vi "SaveTCInfo.vi"(8 "error in (no error)":errorcluster, 10 "Save":bool=TRUE, 11 "TestSeqClass.lvclass":refnum<class "TestSeqClass.lvclass">) -> (0 "error out":errorcluster, 3 "TestSeqClass out":refnum<class "TestSeqClass.lvclass">)   [LabVIEW 2017, in "TestSeqClass.lvclass"]
uses:
  TestSeqClass.lvclass
  Typedef/TestTypeSelect.ctl
  TestMeasureStep/TypeDef/TesstepType.ctl
  Typedef/TestStatus.ctl
  TestMeasureStep/TestMeasureStep.lvclass
  TestMeasureStep/TestMeasureStep.lvclass/TestMeasureStep.ctl
  GUIHandler_Main/GUI_Handler_Main.lvclass
  GUIHandler/GUI_Handler_Seq.lvclass
panel:
  in  "TestType":T1
  in  "ResultListBox":i32(listbox)=-1
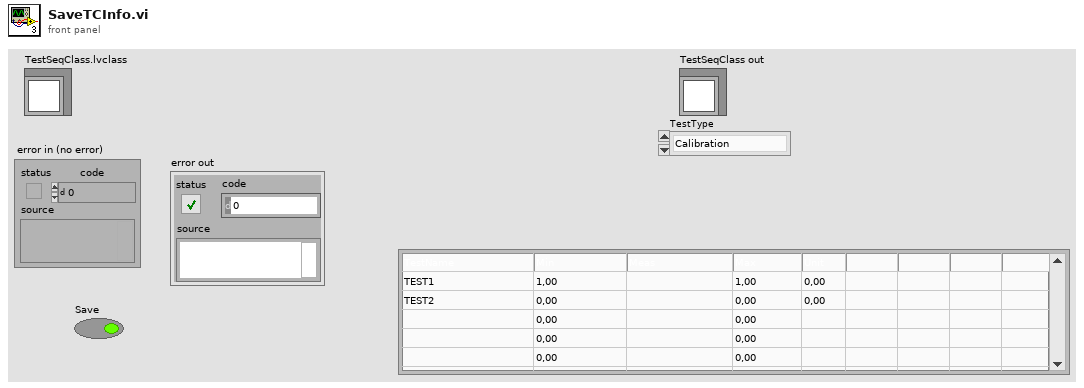
[diagram p1: front panel]
types:
  T1 = typedef "TestTypeSelect.ctl" = enum16{"Calibration", "Testing"}
  T2 = typedef "TestSeqClass.lvclass/TesstepType.ctl" = cluster{"TestName":string, "Meas":dbl, "Min ":dbl, "Max":dbl, "TestStatus":T3, "StringLimit":string, "StringMeas":string, "Unit":string}
  T3 = typedef "TestStatus.ctl" = enum16{"Not Executed", "Passed", "Failed", "Inconclusive", "Processing"}
  T4 = typedef "TestSeqType.ctl" = refnum<class "TestMeasureStep.lvclass">[]
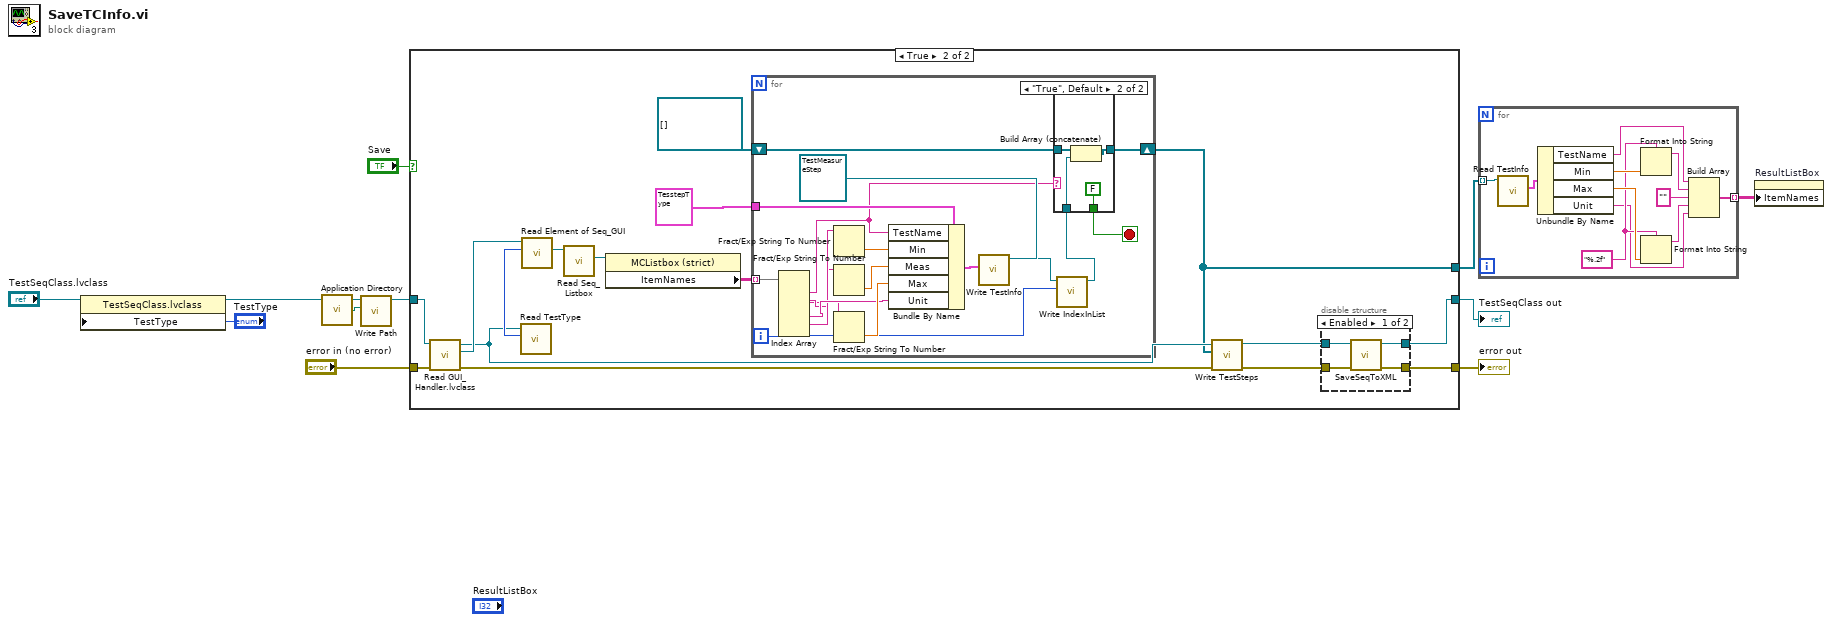
[diagram p0: block diagram]
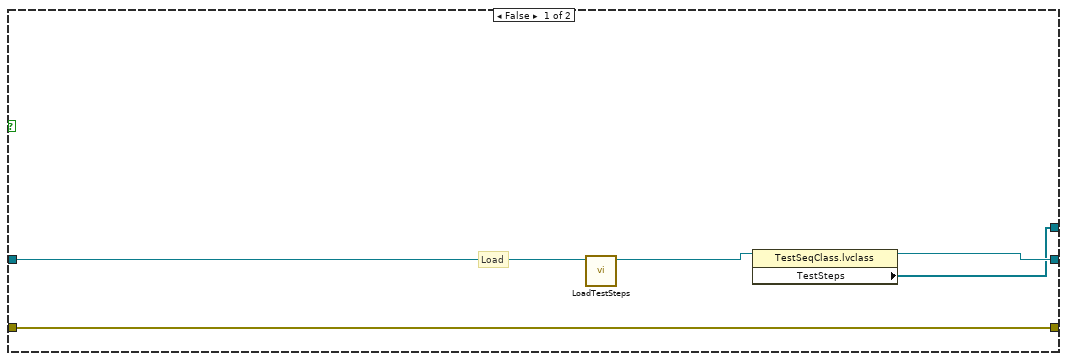
[diagram p2: hidden frame]
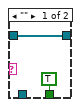
[diagram p4: hidden frame]
diagram:
  n1 = property class="TestSeqClass.lvclass"(reference="TestSeqClass.lvclass", "TestType"="TestType") -> (reference out=w2:refnum<class "TestSeqClass.lvclass">)  [unwired: 1 in, 1 out]
  n2 = call <vilib>:"Application Directory.vi"() -> ("Application Directory"=w5:path)
  n3 = call-dynamic "Write Path.vi"("Path"=w5, "TestSeqClass in"=w2) -> ("TestSeqClass out"=w4:refnum<class "TestSeqClass.lvclass">)  [unwired: 8 in, 1 out]
  n4 = case shown="True" "Save" {
    tunnel: [w16 w31] -> w11
    tunnel: "error in (no error)" -> [w16 w29]
    tunnel: w4 -> [w15 w30]
    tunnel: [w13 w32] -> w7
    tunnel: [w12 w17] -> w6
    frame False {
      # "Load"
      n5 = call-dynamic "LoadTestSteps.vi"("TestSeqClass in"=w15) -> ("TestSeqClass out"=w14:refnum<class "TestSeqClass.lvclass">)  [unwired: 9 in, 1 out]
      n6 = property class="TestSeqClass.lvclass"(reference=w14) -> (reference out=w13:refnum<class "TestSeqClass.lvclass">, "TestSteps"=w12:T4)  [unwired: 1 in, 1 out]
    }
    frame True {
      n7 = call-dynamic "Read GUI_Handler.lvclass.vi"("error in (no error)"=w29, "TestSeqClass in"=w30) -> ("error out"=w19:errorcluster, "GUI_Handler.lvclass"=w25:refnum<class "GUI_Handler_Main.lvclass">, "TestSeqClass out"=w22:refnum<class "TestSeqClass.lvclass">)  [unwired: 7 in]
      n8 = call-dynamic "Read TestType.vi"("TestSeqClass in"=w22) -> ("TestType"=w26:T1)  [unwired: 8 in, 2 out]
      n9 = call-dynamic "Read Element of Seq_GUI.vi"("Variant"=w26, "GUI_Handler_Main in"=w25) -> ("GUI_Handler_Seq.lvclass"=w24:refnum<class "GUI_Handler_Seq.lvclass">)  [unwired: 7 in, 2 out]
      n10 = call-dynamic "Read Seq_Listbox.vi"("GUI_Handler_Seq in"=w24) -> ("Seq_Listbox"=w27:refnum<vi>)  [unwired: 8 in, 2 out]
      n11 = property class="MCListbox (strict)"(reference=w27) -> ("ItemNames"=w28:string[][])  [unwired: 1 in, 2 out]
      n12 = for {
        tunnel: w28 -> [w56] mode=indexing
        tunnel: T2 {"TestName"="", "Meas"=0.0, "Min "=0.0, "Max"=0.0, "TestStatus"=enum."Not Executed", "StringLimit"="", "StringMeas"="", "Unit"=""} ("TestInfo 2") -> [w52]
        shift-right: [w42] -> w17
        shift-left: refnum<class "TestMeasureStep.lvclass">[] [] -> [w41]
        i -> [w48]
        stop <- w39 stop-if-true
        n13 = Index Array(array=w56) -> (element #1=w43:string, element #2=w45:string, element #4=w47:string, element #5=w46:string, element #6=w44:string)  [unwired: 6 in, 1 out]
        n14 = Fract/Exp String To Number(string=w46) -> (number=w55:dbl)  [unwired: 3 in, 1 out]
        n15 = Fract/Exp String To Number(string=w45) -> (number=w54:dbl)  [unwired: 3 in, 1 out]
        n16 = Fract/Exp String To Number(string=w44) -> (number=w53:dbl)  [unwired: 3 in, 1 out]
        n17 = Bundle By Name(cluster=w52, "TestName"=w43, "Min"=w55, "Meas"=w54, "Max"=w53, "Unit"=w47) -> (w51:T2)
        n18 = call-dynamic "Write TestInfo.vi"("TestInfo 2"=w51, "TestMeasureStep in"=refnum<class "TestMeasureStep.lvclass"> refnum ("TestMeasureStep.lvclass")) -> ("TestMeasureStep out"=w49:refnum<class "TestMeasureStep.lvclass">)  [unwired: 8 in, 1 out]
        n19 = call "Write IndexInList.vi"("TestNum"=w48, "TestMeasureStep in"=w49) -> ("TestMeasureStep out"=w40:refnum<class "TestMeasureStep.lvclass">)  [unwired: 8 in, 1 out]
        n20 = case shown="\"True\", Default" w43 {
          tunnel: [w58 w62] -> w42
          tunnel: w41 -> [w58 w61]
          tunnel: w40 -> [_ w60]
          tunnel: [TRUE FALSE] -> w39
          frame "" {
          }
          frame "True", Default {
            n21 = Build Array (concatenate)(w61, w60) -> (w62:refnum<class "TestMeasureStep.lvclass">[])
          }
        }
      }
      n22 = call-dynamic "Write TestSteps.vi"("error in (no error)"=w19, "TestSteps"=w17, "TestSeqClass in"=w22) -> ("error out"=w20:errorcluster, "TestSeqClass out"=w21:refnum<class "TestSeqClass.lvclass">)  [unwired: 7 in]
      n23 = disable-structure shown="Enabled" {
        disable-tunnel: [w36 w38] -> w32
        disable-tunnel: w21 -> [w35 w38]
        disable-tunnel: w20 -> [w34 w37]
        disable-tunnel: [w33 w37] -> w31
        frame Enabled {
          n24 = call-dynamic "SaveSeqToXML.vi"("error in (no error)"=w34, "TestSeqClass in"=w35) -> ("error out"=w33:errorcluster, "TestSeqClass out"=w36:refnum<class "TestSeqClass.lvclass">)  [unwired: 8 in]
        }
        frame Disabled {
        }
      }
    }
  }
  "error out" <- w11
  "TestSeqClass out" <- w7
  n25 = for {
    tunnel: [w73] -> w8 mode=indexing
    tunnel: w6 -> [w64] mode=indexing
    w66 = "%.2f" ("format string")
    n26 = call-dynamic "Read TestInfo.vi"("TestMeasureStep in"=w64) -> ("TestInfo 2"=w63:T2)  [unwired: 8 in, 2 out]
    n27 = Unbundle By Name(w63) -> ("TestName"=w72:string, "Min"=w70:dbl, "Max"=w68:dbl, "Unit"=w65:string)
    n28 = Format Into String(format string=w66, w70) -> (resulting string=w69:string)  [unwired: 2 in, 1 out]
    n29 = Format Into String(format string=w66, w68) -> (resulting string=w67:string)  [unwired: 2 in, 1 out]
    n30 = Build Array(w72, w69, "" ("element"), w67, w65) -> (w73:string[])
  }
  n31 = property on="ResultListBox" class="MCListbox (strict)"("ItemNames"=w8) -> ()  [unwired: 2 in, 2 out]
